vi "Receive.vi"(11 "Base Event in":refnum<class "Base Event.lvclass">) -> (2 "Registration":refnum<event-registration>, 3 "Base Event out":refnum<class "Base Event.lvclass">)   [LabVIEW 2021, in "jettl.lvlib" / "Base Event.lvlib" / "Base Event.lvclass"]
uses:
  Base Event.lvclass
  Msg Strategy/Msg Strategy.lvclass
  Base Event.lvclass/Base Event.ctl
  Self Event/Self Event.lvlib
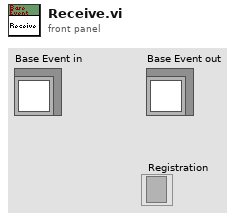
[diagram p1: front panel]
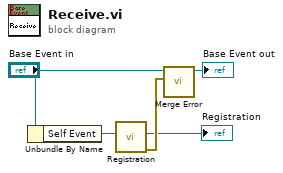
[diagram p0: block diagram]
diagram:
  n1 = Unbundle By Name("Base Event in") -> ("Self Event"=w2:refnum<data-value>)
  n2 = call "Registration.vi"("Self Event"=w2) -> ("error out"=w3:errorcluster, "Registration"=→"Registration":refnum<event-registration>)  [unwired: 9 in]
  n3 = call-dynamic "Merge Error.vi"("Error"=w3, "Base Event in"="Base Event in") -> ("Base Event out"=→"Base Event out":refnum<class "Base Event.lvclass">)  [unwired: 9 in]
